vi "power read.vi"(7 "Max Voltage":dbl=8.5 format="%.2f", 11 "error in (no error)":errorcluster) -> (8 "normalized Power Read (0-1)":dbl=0.0244140625 format="%.2f", 15 "error out":errorcluster)   [LabVIEW 2016]
doc: "This one shot VI reads the power in via analog in. The voltage is measured and converted to a normalized power.\n\nPaul K Dixon\nPhysics 350\nPaul K Dixon"
panel:
  in  "channel (0)":tag="Dev1/ai0"
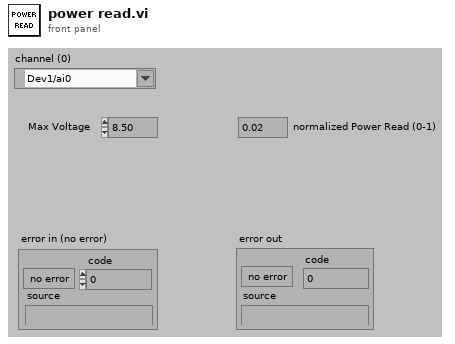
[diagram p1: front panel]
types:
  T1 = enum16{"AI sample channel scan", "AI Waveform triggered"}
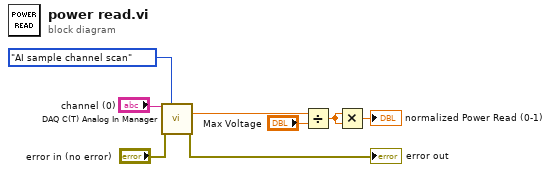
[diagram p0: block diagram]
diagram:
  n1 = call "DAQ C(T) Analog In Manager.vi"("channel (single point) (0)"="channel (0)", "AI mode chooser"=T1."AI sample channel scan", "error in (no error)"="error in (no error)") -> ("V meas"=w2:dbl, "error out"=→"error out":errorcluster)  [unwired: 5 in, 6 out]
  n2 = Divide(x=w2, y="Max Voltage") -> (x/y=w6:dbl)
  n3 = Multiply(x=w6, y=w6) -> (x*y=→"normalized Power Read (0-1)":dbl)
